vi "Stufen abfragen Tabelle setzen und auslesen.vi"(4 "E/A Cluster":T4, 5 "Ausgabetabelle (Eingang)":refnum<vi>, 6 "GD Cluster":T3, 7 "Eingabetabelle (Eingang)":refnum<vi>, 8 "Fehler (Eingang, kein Fehler)":errorcluster, 9 "Komponente in":T7, 10 "Index Cluster":T1, 11 "GD in":T6) -> (0 "Fehler (Ausgang)":errorcluster, 1 "Komponente out":T7, 2 "EGAK out":T5[](array[typedef]), 3 "Stufen Tabellen out":string[][](array[string]))   [LabVIEW 2020, in "Linearisierung v2.lvlib" / "SpanEinstellungen.lvlib"]
uses:
  SpanEinstellungen.lvlib
  Visualisierungs Elemente/Auswahlfeld.ctl
  Seiten/System Einstellungen V2/Traegergas.ctl
  Seiten/System Einstellungen V2/Konfig Gasflasche.ctl
  Aktion Lin Daten aufarbeiten.ctl
  Aktion FGV SPAN Stufentabellen.ctl
  Linearisierung v2.lvlib
  Gasteiler/Gasteiler.lvlib
  Seiten/System Einstellungen V2/System Einstellungen V2.lvlib
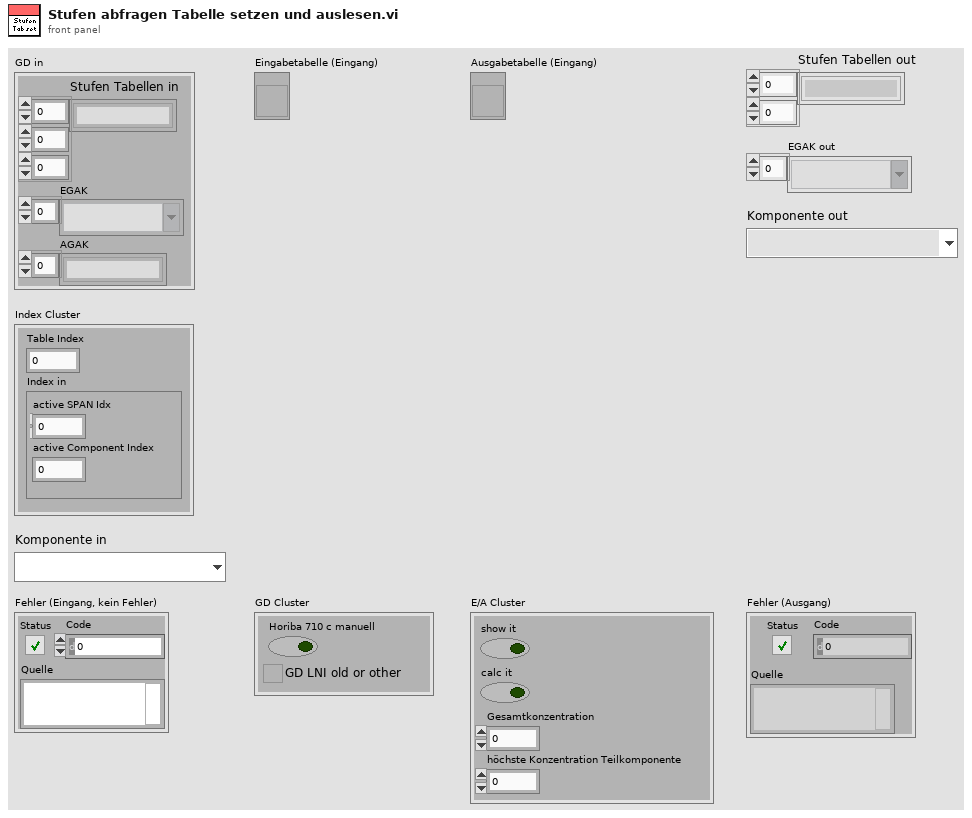
[diagram p1: front panel]
types:
  T1 = cluster{"Table Index":i32, "Index in":cluster{"active SPAN Idx":i32, "active Component Index":i32}}
  T2 = typedef "System Einstellungen V2.lvlib/Konfig Gasflasche.ctl" = bool
  T3 = cluster{"Horiba 710 c manuell":bool, "GD LNI old or other":T2}
  T4 = cluster{"show it":bool, "calc it":bool, "Gesamtkonzentration":dbl, "höchste Konzentration Teilkomponente":dbl}
  T5 = typedef "System Einstellungen V2.lvlib/Traegergas.ctl" = string
  T6 = cluster{"Stufen Tabellen in":string[][][], "EGAK":T5[], "AGAK":string[]}
  T7 = typedef "Auswahlfeld.ctl" = u16
  T8 = typedef "Linearisierung v2.lvlib/SpanEinstellungen.lvlib/Aktion FGV SPAN Stufentabellen.ctl" = enum16{"lesen", "schreiben", "init"}
  T9 = typedef "Linearisierung v2.lvlib/Aktion Lin Daten aufarbeiten.ctl" = enum16{"lesen", "Protkolldaten", "speichern", "laden", "EPA auswerten", "Tabelle schreiben", "Lin auswerten", "Tab init", "Stufentabelle", "EPA aktiviert", "Nachbehandlung laden", "Tabelle löschen", "Istwerte löschen", "Zeile löschen", "Zeile einfügen", "LIN aktiviert", "LIN/EPA aktiv laden", "EGAK Tab", "LIN übernehmen", "Tab init ohne Stufen"}
  T10 = cluster{"active SPAN Idx":i32, "active Component Index":i32}
  T11 = typedef "Linearisierung v2.lvlib/Eingabetabelle.ctl" = string[][]
  T12 = typedef "Linearisierung v2.lvlib/Gasteiler.lvlib/Stufen Tabelle.ctl" = string[][]
  T13 = cluster{"active SPAN Idx":i32, "active Component Index":i32, "Stufen Tabellen in":string[][], "EGAK":T5[]}
  T14 = typedef "Linearisierung v2.lvlib/Ausgabetabelle.ctl" = string[][]
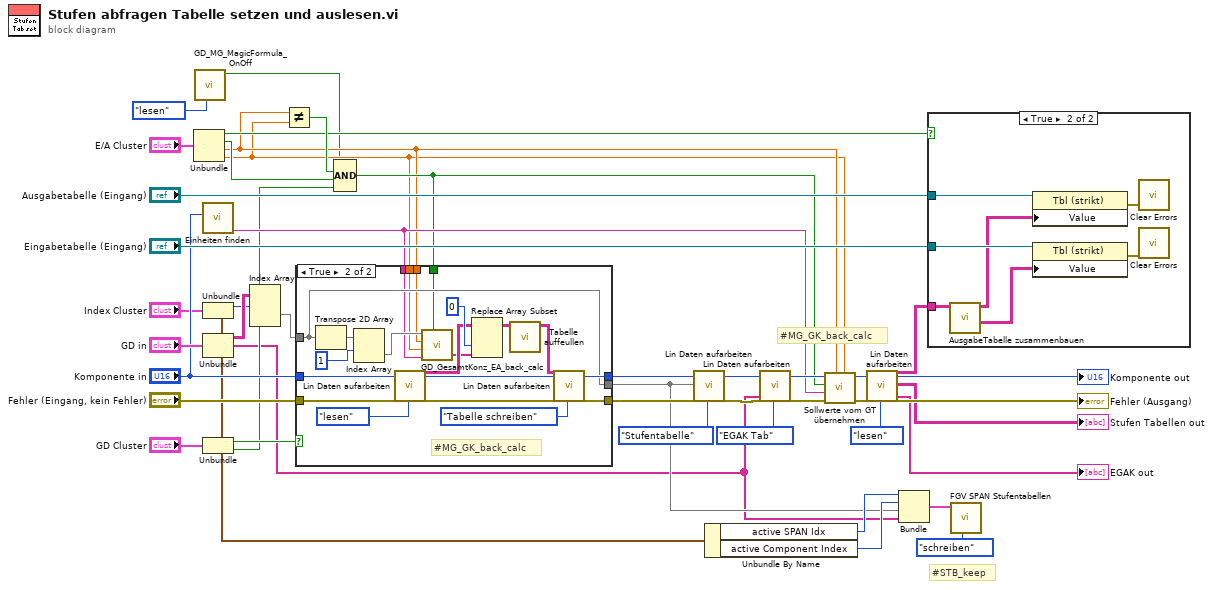
[diagram p0: block diagram]
diagram:
  # "#STB_keep"
  # "#MG_GK_back_calc"
  n1 = Unbundle("E/A Cluster") -> ("show it"=w18:bool, "calc it"=w17:bool, "Gesamtkonzentration"=w16:dbl, "höchste Konzentration Teilkomponente"=w15:dbl)
  n2 = call "GD_MG_MagicFormula_OnOff.vi"("Aktion"=enum16{"lesen", "schreiben", "init"}."lesen") -> ("MG_use_magic_formula"=w11:bool)  [unwired: 8 in, 1 out]
  n3 = call "Einheiten finden.vi"("Komponente"="Komponente in") -> ("Einheit in String"=w20:string)  [unwired: 6 in, 4 out]
  n4 = Unbundle("Index Cluster") -> ("Table Index"=w8:i32, "Index in"=w3:T10)
  n5 = Unbundle("GD in") -> ("Stufen Tabellen in"=w26:string[][][], "EGAK"=w1:T5[])  [unwired: 1 out]
  n6 = Unbundle("GD Cluster") -> ("Horiba 710 c manuell"=w13:bool, "GD LNI old or other"=w12:T2)
  n7 = Index Array(array=w26, index (dim 0)=w8) -> (element=w25:string[][])  [unwired: 2 in]
  n8 = Not Equal?(x=w16, y=w15) -> (x != y?=w21:bool)
  n9 = Compound Arithmetic op=AND ("Mehrfacharithmetik")(w11, w21, w17, w12) -> (w19:T2)
  n10 = case shown="True" w13 {
    tunnel: w25 -> [w46 w57]
    tunnel: "Fehler (Eingang, kein Fehler)" -> [w47 w61]
    tunnel: [w47 w59] -> w38
    tunnel: "Komponente in" -> [w48 w56]
    tunnel: [w48 w58] -> w45
    tunnel: [w46 w57] -> w2
    tunnel: w20 -> [_ w49]
    tunnel: w19 -> [_ w52]
    tunnel: w16 -> [_ w51]
    tunnel: w15 -> [_ w50]
    frame False {
    }
    frame True {
      # "#MG_GK_back_calc"
      n11 = Transpose 2D Array(2D array=w57) -> (transposed array=w63:string[][])
      n12 = Index Array(array=w63, index (row)=1 ("Index (Zeile)")) -> (element=w53:string[])  [unwired: 1 in]
      n13 = call "Lin Daten aufarbeiten.vi"("Index (Seite)"=w56, "error in (no error)"=w61, "Aktionen"=Aktion_Lin_Daten_aufarbeiten."lesen") -> ("Eingabetabelle"=w65:T11, "Index (Seite) out"=w55:i32, "error out"=w60:errorcluster)  [unwired: 14 in, 8 out]
      n14 = call "GD_GesamtKonz_EA_back_calc.vi"("DoIt"=w52, "Einheit in String"=w49, "höchste Konzentration Teilkomponente"=w50, "Gesamtkonzentration"=w51, "Stufentabelle (Eingang)"=w53) -> ("Sollwerte EA Tabelle (Ausgang)"=w54:string[])  [unwired: 6 in]
      n15 = Replace Array Subset(array=w65, new element=w54, index (col)=0 ("Deaktivierter Index (Spalte)")) -> (w68:T11)  [unwired: 1 in]
      n16 = call "Tabelle auffeullen.vi"("Neue Tabelle"=w68) -> ("Tabelle"=w69:string[][])  [unwired: 10 in]
      n17 = call "Lin Daten aufarbeiten.vi"("Eingabetabelle"=w69, "Index (Seite)"=w55, "error in (no error)"=w60, "Aktionen"=Aktion_Lin_Daten_aufarbeiten."Tabelle schreiben") -> ("Index (Seite) out"=w58:i32, "error out"=w59:errorcluster)  [unwired: 13 in, 9 out]
    }
  }
  n18 = call "Lin Daten aufarbeiten.vi"("Index (Seite)"=w45, "Stufen Tabelle"=w2, "error in (no error)"=w38, "Aktionen"=Aktion_Lin_Daten_aufarbeiten."Stufentabelle") -> ("Index (Seite) out"=w43:i32, "error out"=w36:errorcluster)  [unwired: 13 in, 9 out]
  n19 = Unbundle By Name(w3) -> ("active SPAN Idx"=w7:i32, "active Component Index"=w6:i32)
  n20 = call "Lin Daten aufarbeiten.vi"("Index (Seite)"=w43, "EGAK"=w1, "error in (no error)"=w36, "Aktionen"=Aktion_Lin_Daten_aufarbeiten."EGAK Tab") -> ("Index (Seite) out"=w32:i32, "error out"=w30:errorcluster)  [unwired: 13 in, 9 out]
  n21 = call "Sollwerte vom GT übernehmen.vi"("höchste Konzentration Teilkomponente"=w15, "Gesamtkonzentration"=w16, "error in (no error)"=w30, "Einheit in String"=w20, "DoIt"=w19, "Gasindex"=w32) -> ("error out"=w29:errorcluster, "Gasindex out"=w31:i32)  [unwired: 4 in]
  n22 = call "Lin Daten aufarbeiten.vi"("Index (Seite)"=w31, "error in (no error)"=w29, "Aktionen"=Aktion_Lin_Daten_aufarbeiten."lesen") -> ("Eingabetabelle"=w34:T11, "Index (Seite) out"=→"Komponente out":i32, "Stufen Tabelle"=→"Stufen Tabellen out":T12, "EKAG"=→"EGAK out":string[], "error out"=→"Fehler (Ausgang)":errorcluster)  [unwired: 14 in, 6 out]
  n23 = Bundle("active SPAN Idx"=w7, "active Component Index"=w6, "Stufen Tabellen in"=w2, "EGAK"=w1) -> (w4:T13)  [unwired: 1 in]
  n24 = case shown="True" w18 {
    tunnel: "Eingabetabelle (Eingang)" -> [_ w76]
    tunnel: w34 -> [_ w74]
    tunnel: "Ausgabetabelle (Eingang)" -> [_ w72]
    frame False {
    }
    frame True {
      n25 = call "AusgabeTabelle zusammenbauen.vi"("Eingabetabelle"=w74) -> ("Eingabetabelle behandelt"=w73:string[][], "Ausgabetabelle"=w71:T14)  [unwired: 8 in, 1 out]
      n26 = property class="Tbl (strikt)"(reference=w72, "Value"=w71) -> (error out=w70:errorcluster)  [unwired: 1 in, 1 out]
      n27 = property class="Tbl (strikt)"(reference=w76, "Value"=w73) -> (error out=w75:errorcluster)  [unwired: 1 in, 1 out]
      n28 = call <vilib>:"Clear Errors.vi"("error in (no error)"=w70) -> ()  [unwired: 5 in, 2 out]
      n29 = call <vilib>:"Clear Errors.vi"("error in (no error)"=w75) -> ()  [unwired: 5 in, 2 out]
    }
  }
  n30 = call "FGV SPAN Stufentabellen.vi"("Aktion"=Aktion_FGV_SPAN_Stufentabellen."schreiben", "In Cluster"=w4) -> ()  [unwired: 5 in, 4 out]
